vi "AutoTargetTeleop.vi"   [LabVIEW 2015]
uses:
  VisionGlobals.vi
  GeneralGlobals.vi
  GlobalVisionVars.vi
  MotorPositionGlobals.vi
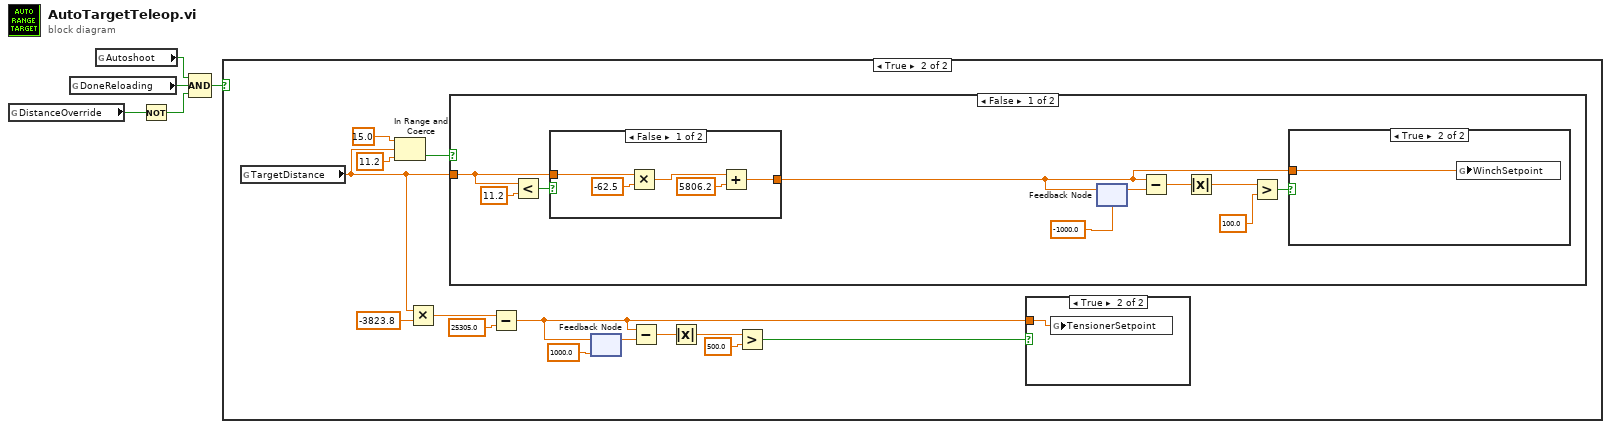
[diagram p0: block diagram]
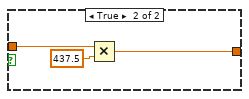
[diagram p3: hidden frame]
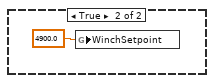
[diagram p5: hidden frame]
diagram:
  n1 = global read "GeneralGlobals.vi" "DistanceOverride"() -> (w2:bool)
  n2 = global read "GeneralGlobals.vi" "DoneReloading"() -> (w4:bool)
  n3 = global read "VisionGlobals.vi" "Autoshoot"() -> (w5:bool)
  n4 = Not(x=w2) -> (.not. x?=w1:bool)
  n5 = Compound Arithmetic op=AND(w5, w4, w1) -> (w3:bool)
  n6 = case shown="True" w3 {
    frame False {
    }
    frame True {
      n7 = global read "GlobalVisionVars.vi" "TargetDistance"() -> (w6:dbl)
      n8 = In Range and Coerce(upper limit=15.0, x=w6, lower limit=11.2) -> (In Range?=w7:bool)  [unwired: 1 out]
      n9 = Multiply(x=w6, y=-3823.8) -> (x*y=w18:dbl)
      n10 = case shown="False" w7 {
        tunnel: w6 -> [w21 _]
        frame False {
          n11 = Less?(x=w21, y=11.2) -> (x < y?=w23:bool)
          n12 = case shown="False" w23 {
            tunnel: w21 -> [w33 w37]
            tunnel: [w32 w35] -> w20
            frame False {
              n13 = Multiply(x=w33, y=-62.5) -> (x*y=w31:dbl)
              n14 = Add(x=w31, y=5806.2) -> (x+y=w32:dbl)
            }
            frame True {
              n15 = Multiply(x=w37, y=437.5) -> (x*y=w35:dbl)
            }
          }
          n16 = feedback #1(-1000.0) -> (w29:dbl)
          n17 = feedback-in #1(w20) -> ()
          n18 = Subtract(x=w20, y=w29) -> (x-y=w27:dbl)
          n19 = Absolute Value(x=w27) -> (abs(x)=w26:dbl)
          n20 = Greater?(x=w26, y=100.0) -> (0:w24:bool)
          n21 = case shown="True" w24 {
            tunnel: w20 -> [_ w38]
            frame False {
            }
            frame True {
              n22 = global write "MotorPositionGlobals.vi" "WinchSetpoint"(w38) -> ()
            }
          }
        }
        frame True {
          n23 = global write "MotorPositionGlobals.vi" "WinchSetpoint"(4900.0 ("WinchSetpoint")) -> ()
        }
      }
      n24 = Subtract(x=w18, y=25305.0) -> (x-y=w16:dbl)
      n25 = feedback #2(1000.0) -> (w15:dbl)
      n26 = feedback-in #2(w16) -> ()
      n27 = Subtract(x=w16, y=w15) -> (x-y=w13:dbl)
      n28 = Absolute Value(x=w13) -> (abs(x)=w12:dbl)
      n29 = Greater?(x=w12, y=500.0) -> (0:w10:bool)
      n30 = case shown="True" w10 {
        tunnel: w16 -> [_ w40]
        frame False {
        }
        frame True {
          n31 = global write "MotorPositionGlobals.vi" "TensionerSetpoint"(w40) -> ()
        }
      }
    }
  }
